vi "Create Image Array.vi"(0 "# of imgs":i32, 2 "Border Size":i32=3, 7 "Image Array Base Name":string="Buffer", 11 "error in (no error)":errorcluster, 13 "Image Type":T1 items=["Grayscale (U8)", "Grayscale (I16)", "Grayscale (SGL)", "Complex (CSG)", "RGB (U32)", "HSL (U32)", "RGB (U64)"]) -> (4 "Img Array":T2[](array[typedef]), 15 "error out":errorcluster)   [LabVIEW 2013]
uses:
  <vilib>/vision/Image Controls.llb/IMAQ Image.ctl
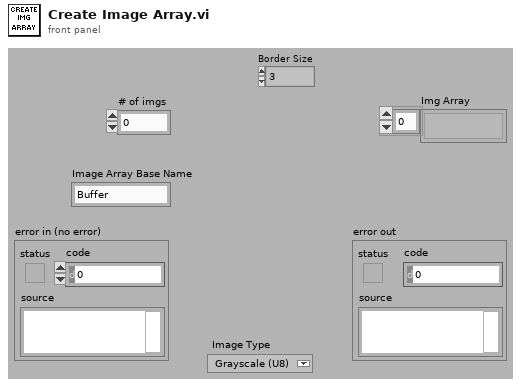
[diagram p1: front panel]
types:
  T1 = typedef "Image Type" = u32
  T2 = typedef "IMAQ Image.ctl" = refnum<image>
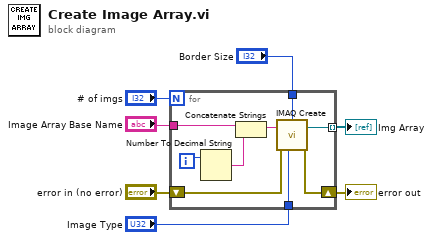
[diagram p0: block diagram]
diagram:
  n1 = for {
    N: "# of imgs" -> [_]
    tunnel: [w13] -> w6 mode=indexing
    tunnel: "Image Type" -> [w8]
    tunnel: "Image Array Base Name" -> [w12]
    shift-right: [w10] -> w4
    shift-left: "error in (no error)" -> [w11]
    tunnel: "Border Size" -> [w9]
    i -> [w16]
    n2 = Number To Decimal String(number=w16) -> (decimal integer string=w15:string)  [unwired: 1 out]
    n3 = Concatenate Strings(w12, w15) -> (w14:string)
    n4 = call "IMAQ Create"("Border Size"=w9, "Image Name"=w14, "Image Type"=w8, "error in (no error)"=w11) -> ("New Image"=w13:T2, "error out"=w10:errorcluster)  [unwired: 1 out]
  }
  "Img Array" <- w6
  "error out" <- w4
